vi "Node - Config Reader.vi"(8 "error in (no error)":errorcluster, 11 "Node Data In":T1) -> (0 "error out":errorcluster, 3 "Node Data Out":T1)   [LabVIEW 2016, in "PXImc Router.lvlib"]
uses:
  PXImc Router.lvlib
  Controls/Node/Node - Config.ctl
  <vilib>/NI Veristand/VeriStand Data/Byte Buffer/Byte Buffer.lvclass
  Controls/Node/Node - PXImc Parameters.ctl
  Controls/Node/Node - Writer Data.ctl
  Controls/Node/Node - Ch Properties.ctl
  Controls/Data Type.ctl
  Controls/Node/Node - Readers Data.ctl
  Controls/Node/Node - Reader Data.ctl
  <vilib>/NI Veristand/VeriStand Data/Byte Buffer/Byte Buffer.lvclass/Byte Buffer.ctl
  <vilib>/NI Veristand/VeriStand Data/Byte Buffer/Byte Buffer.Get Buffer Pointer.vi
  <vilib>/NI Veristand/VeriStand Data/Byte Buffer/Byte Buffer.Get Buffer Size.vi
  <vilib>/NI Veristand/VeriStand Data/Memory Management/Memory Management.MoveByteBlock (Pointer).vi
  <vilib>/NI Veristand/VeriStand Data/Pointer Operations/Pointer.New.vi
  <vilib>/NI Veristand/VeriStand Data/Pointer Operations/Pointer.Dispose.vi
  <vilib>/NI Veristand/VeriStand Data/Byte Buffer/Byte Buffer.Set Buffer Pointer.vi
  <vilib>/NI Veristand/VeriStand Data/Byte Buffer/Byte Buffer.Set Buffer Size.vi
  <vilib>/NI Veristand/VeriStand Data/Memory Management/Memory Management.Handle Return.vi
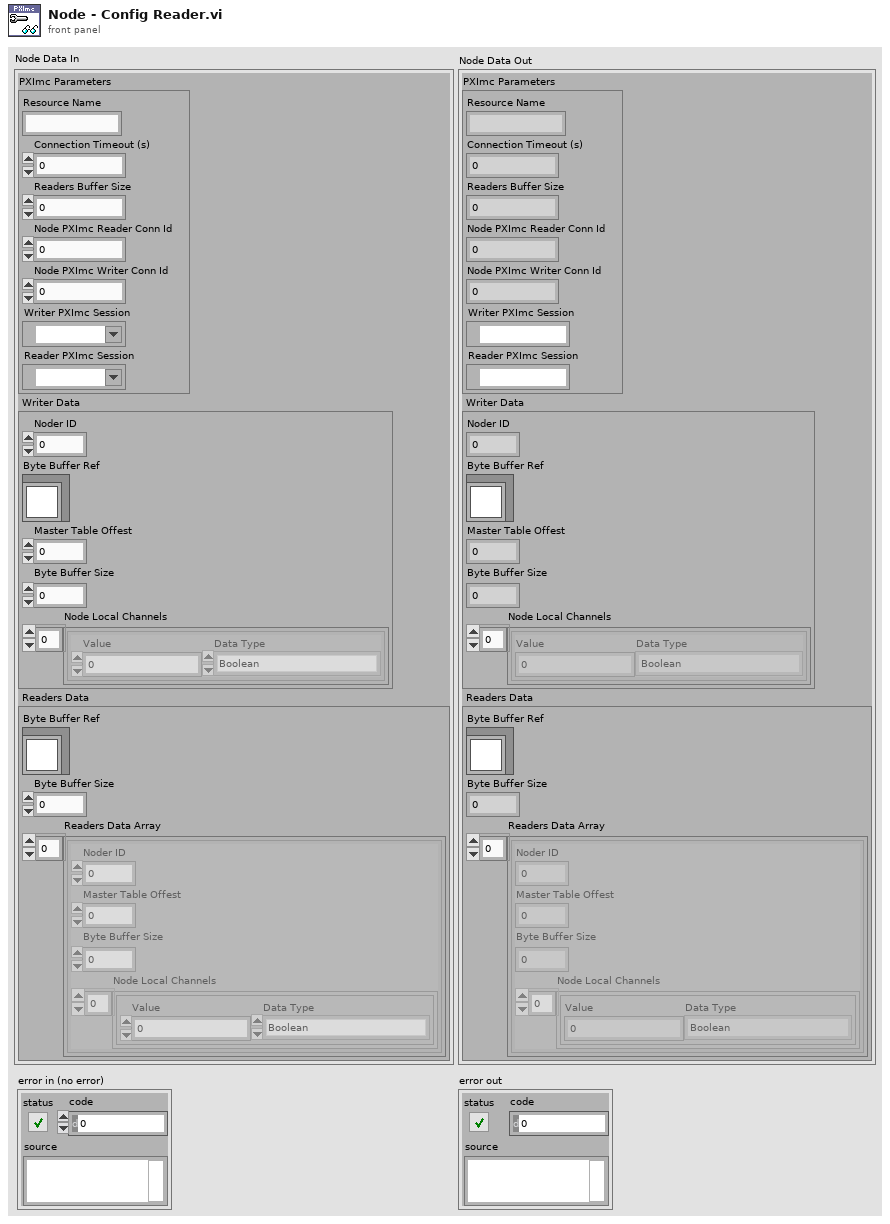
[diagram p1: front panel]
types:
  T1 = typedef "PXImc Router.lvlib/Node - Config.ctl" = cluster{"PXImc Parameters":T2, "Writer Data":T3, "Readers Data":T6}
  T2 = typedef "PXImc Router.lvlib/Node - PXImc Parameters.ctl" = cluster{"Resource Name":string, "Connection Timeout (s)":dbl, "Readers Buffer Size":u64, "Node PXImc Reader Conn Id":u16, "Node PXImc Writer Conn Id":u16, "Writer PXImc Session":refnum<k21>, "Reader PXImc Session":refnum<k21>}
  T3 = typedef "PXImc Router.lvlib/Node - Writer Data.ctl" = cluster{"Noder ID":u32, "Byte Buffer Ref":refnum<class "Byte Buffer.lvclass">, "Master Table Offest":u32, "Byte Buffer Size":u32, "Node Local Channels":T4[]}
  T4 = typedef "PXImc Router.lvlib/Node - Ch Properties.ctl" = cluster{"Value":dbl, "Data Type":T5}
  T5 = typedef "PXImc Router.lvlib/Data Type.ctl" = enum16{"Boolean", "SGL", "DBL", "I8", "I16", "I32", "I64", "U8", "U16", "U32", "U64"}
  T6 = typedef "PXImc Router.lvlib/Node - Readers Data.ctl" = cluster{"Byte Buffer Ref":refnum<class "Byte Buffer.lvclass">, "Byte Buffer Size":u64, "Readers Data Array":T7[]}
  T7 = typedef "PXImc Router.lvlib/Node - Reader Data.ctl" = cluster{"Noder ID":u32, "Master Table Offest":u32, "Byte Buffer Size":u64, "Node Local Channels":T4[]}
  T8 = typedef "PXImc Router.lvlib/Node - Buffer Offsets - Indexes.ctl" = cluster{"Buffer Offsets":u64, "Indexes":i32}
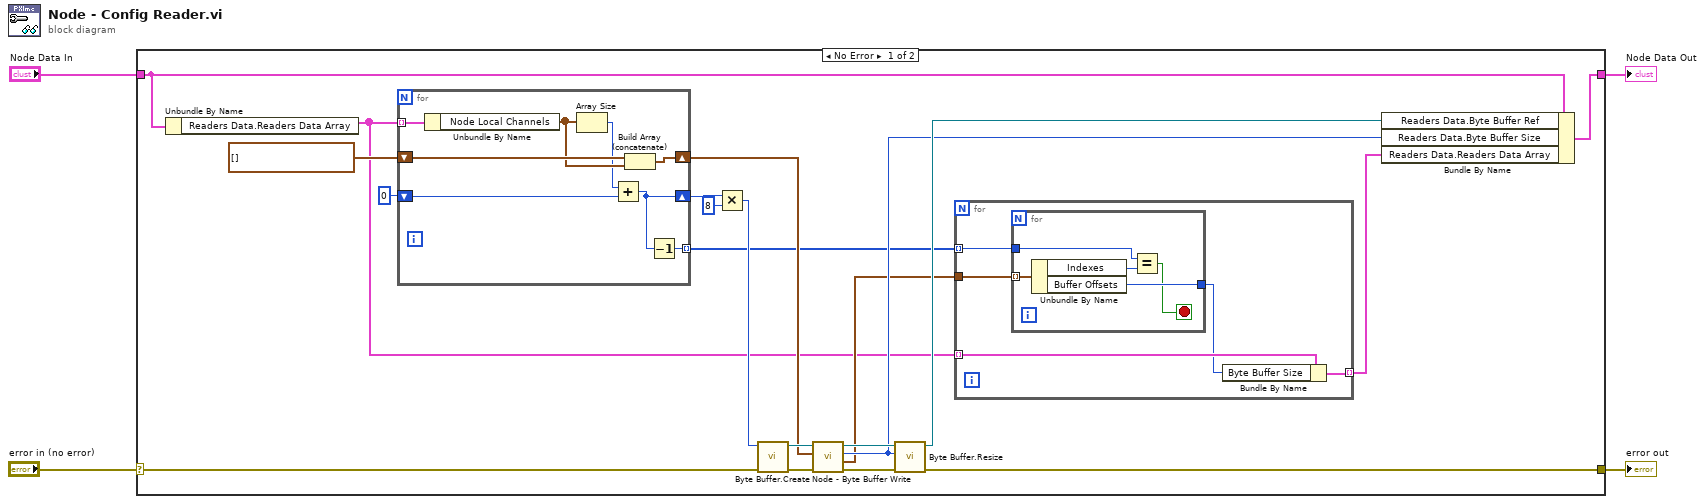
[diagram p0: block diagram]
diagram:
  n1 = case shown="No Error" "error in (no error)" {
    selector: "error in (no error)" -> [w18 w44]
    tunnel: [w24 w43] -> w4
    tunnel: [w12 w44] -> w3
    tunnel: "Node Data In" -> [w7 w43]
    frame No Error {
      n2 = Unbundle By Name(w7) -> ("Readers Data.Readers Data Array"=w6:T7[])
      n3 = for {
        tunnel: w6 -> [w42] mode=indexing
        shift-right: [w36] -> w11
        shift-left: 0 ("x*y") -> [w41]
        shift-right: [w38] -> w15
        shift-left: T4[] [] ("Node Local Channels") -> [w40]
        tunnel: [w35] -> w9 mode=indexing
        n4 = Unbundle By Name(w42) -> ("Node Local Channels"=w39:T4[])
        n5 = Array Size(array=w39) -> (size(s)=w37:i32)
        n6 = Add(x=w37, y=w41) -> (x+y=w36:i32)
        n7 = Build Array (concatenate)(w40, w39) -> (w38:T4[])
        n8 = Decrement(x=w36) -> (x-1=w35:i32)
      }
      n9 = Multiply(x=w11, y=8) -> (x*y=w17:i32)
      n10 = call <vilib>:"Byte Buffer.Create.vi"("error in (no error)"=w18, "size"=w17) -> ("error out"=w19:errorcluster, "Byte Buffer"=w16:refnum<class "Byte Buffer.lvclass">)  [unwired: 8 in]
      n11 = call "Node - Byte Buffer Write.vi"("error in (no error)"=w19, "Node Local Channels"=w15, "Byte Buffer In"=w16) -> ("error out"=w20:errorcluster, "Buffer Offsets - Indexes Out"=w8:T8[], "Buffer Offset Out"=w13:u64, "Byte Buffer Out"=w21:refnum<class "Byte Buffer.lvclass">)  [unwired: 5 in]
      n12 = call <vilib>:"Byte Buffer.Resize.vi"("error in (no error)"=w20, "new size"=w13, "Byte Buffer in"=w21) -> ("error out"=w12:errorcluster, "Byte Buffer out"=w14:refnum<class "Byte Buffer.lvclass">)  [unwired: 7 in]
      n13 = for {
        tunnel: w9 -> [w28] mode=indexing
        tunnel: w8 -> [w29]
        tunnel: w6 -> [w27] mode=indexing
        tunnel: [w25] -> w5 mode=indexing
        n14 = for {
          tunnel: w29 -> [w34] mode=indexing
          tunnel: w28 -> [w32]
          tunnel: [w31] -> w26
          stop <- w30 stop-if-true
          n15 = Unbundle By Name(w34) -> ("Indexes"=w33:i32, "Buffer Offsets"=w31:u64)
          n16 = Equal?(x=w32, y=w33) -> (x = y?=w30:bool)
        }
        n17 = Bundle By Name(cluster=w27, "Byte Buffer Size"=w26) -> (w25:T7)
      }
      n18 = Bundle By Name(cluster=w7, "Readers Data.Byte Buffer Ref"=w14, "Readers Data.Byte Buffer Size"=w13, "Readers Data.Readers Data Array"=w5) -> (w24:T1)
    }
    frame Error {
    }
  }
  "error out" <- w3
  "Node Data Out" <- w4
